vi "read_db_for_plot.vi"(6 "Small?":bool, 8 "error in (no error)":errorcluster, 9 "Limit no. of events":dbl=10000.0, 10 "Limited?":bool=TRUE, 11 "Constraints":T1 {"Estimate Quality" scale=0.0..5.0}) -> (0 "error out":errorcluster, 1 "Total Number of events":i64, 2 "Matching Events":i64, 3 "Dust Array":T2[](array[typedef]) {"File Location" items=["Unknown"=-5, "IDL Processing"=-4, "Writing from Queue"=-3, "Labview Files"=-2, "Retry Labview files"=-1, "Local Cache "=0, "Storage"=1]; "Estimate Source" items=["Any Source."=-2, "No Shot"=-1, "Basic Labview Estimate"=0, "IDL Estimate From Andrew"=1, "IDL Estimate From Tobin"=2, "Old Metadata"=3]}, 4 "Dust Info":cluster{"Density":dbl, "Name":string}[](array[cluster]))   [LabVIEW 2013]
uses:
  Public API/Query_Dust_Event.ctl
  Controls/Estimate_source.ctl
  Controls/File_location.ctl
  Controls/Constraints.ctl
  <vilib>/addons/database/Auxilliary.llb/DB Tools Cursor Type.ctl
  <userlib>/_OpenG.lib/array/array.llb/Remove Duplicates from 1D Array (String)__ogtk.vi
  <userlib>/_OpenG.lib/array/array.llb/Search 1D Array (String)__ogtk.vi
  <userlib>/_OpenG.lib/array/array.llb/Delete Elements from 1D Array (String)__ogtk.vi
  <vilib>/addons/database/Connection.llb/Conn Execute.vi
  <vilib>/addons/database/Recordset.llb/Rec Fetch Recordset Data (R).vi
  <vilib>/addons/database/Recordset.llb/Rec Destroy - Connection.vi
  <vilib>/addons/database/_DB Variant To Data/Database Variant To Data.xnode
  <vilib>/addons/database/NI_Database_API.lvlib
panel:
  out "Count Matching Events Syntax":string
  out "Count Events Syntax":string
  out "SQL Query Syntax":string
  # "Dust Event"
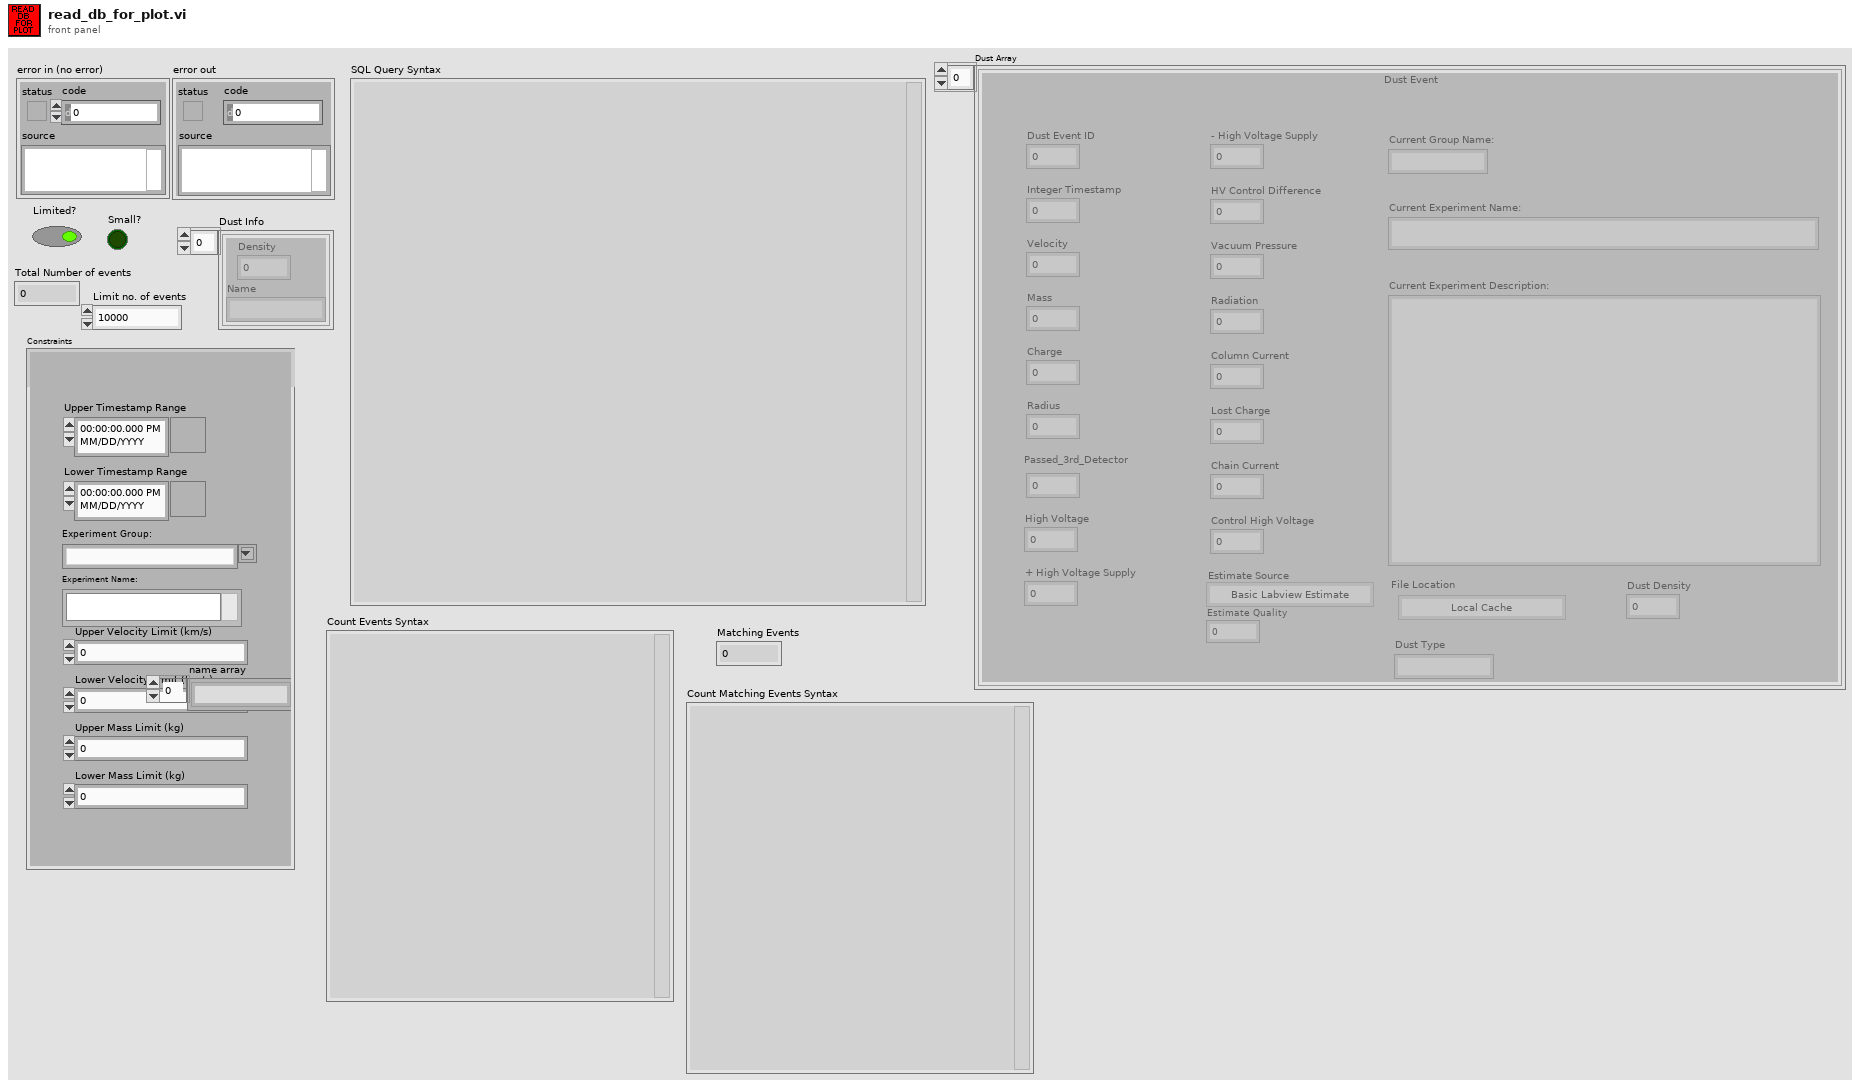
[diagram p1: front panel]
types:
  T1 = typedef "Constraints.ctl" = cluster{"Upper Timestamp Range":timestamp, "Lower Timestamp Range":timestamp, "Experiment Group:":string, "Experiment Name:":i32[], "Upper Velocity Limit (km/s)":dbl, "Lower Velocity Limit (km/s)":dbl, "Upper Mass Limit (kg)":dbl, "Lower Mass Limit (kg)":dbl, "name array":string[], "Estimate Quality":cluster{dbl, dbl}}
  T2 = typedef "Query_Dust_Event.ctl" = cluster{"Dust Event ID":i64, "Integer Timestamp":i64, "Velocity":sgl, "Mass":sgl, "Charge":sgl, "Radius":sgl, "Passed_3rd_Detector":i8, "High Voltage":sgl, "+ High Voltage Supply":sgl, "- High Voltage Supply":sgl, "HV Control Difference":sgl, "Vacuum Pressure":sgl, "Radiation":sgl, "Column Current":sgl, "Lost Charge":sgl, "Chain Current":sgl, "Control High Voltage":sgl, "Current Group Name:":string, "Current Experiment Name:":string, "Current Experiment Description:":string, "Estimate Source":T3, "Estimate Quality":sgl, "File Location":T4, "Dust Type":string, "Dust Density":sgl}
  T3 = typedef "Estimate_source.ctl" = i8
  T4 = typedef "File_location.ctl" = i8
  T5 = typedef "NI_Database_API.lvlib/DB Tools Cursor Type.ctl" = enum16{"forward-only", "keyset", "dynamic", "static"}
  T6 = typedef "NI_Database_API.lvlib/Conn ObjectReference.ctl" = refnum<k1>
  T7 = typedef "NI_Database_API.lvlib/Rec ObjectReference.ctl" = refnum<k1>
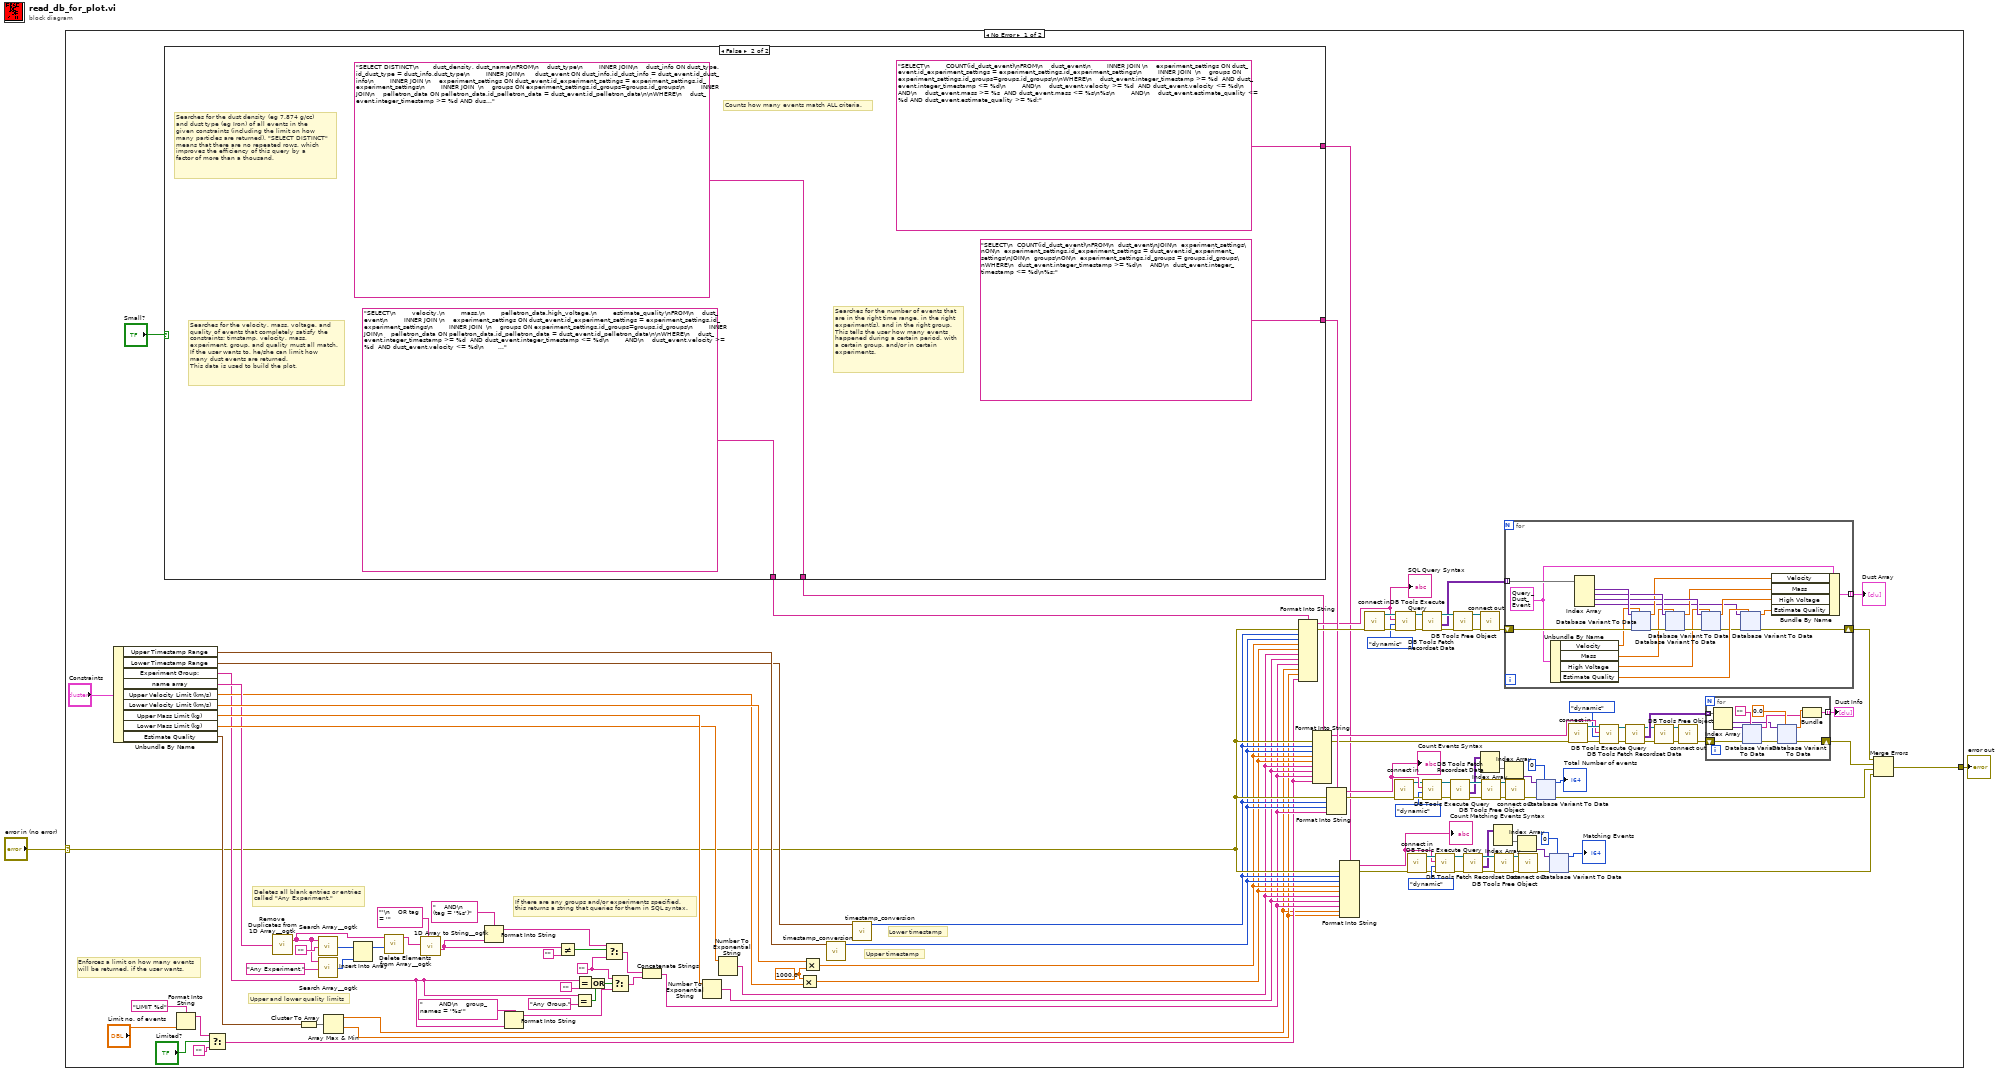
[diagram p0: block diagram]
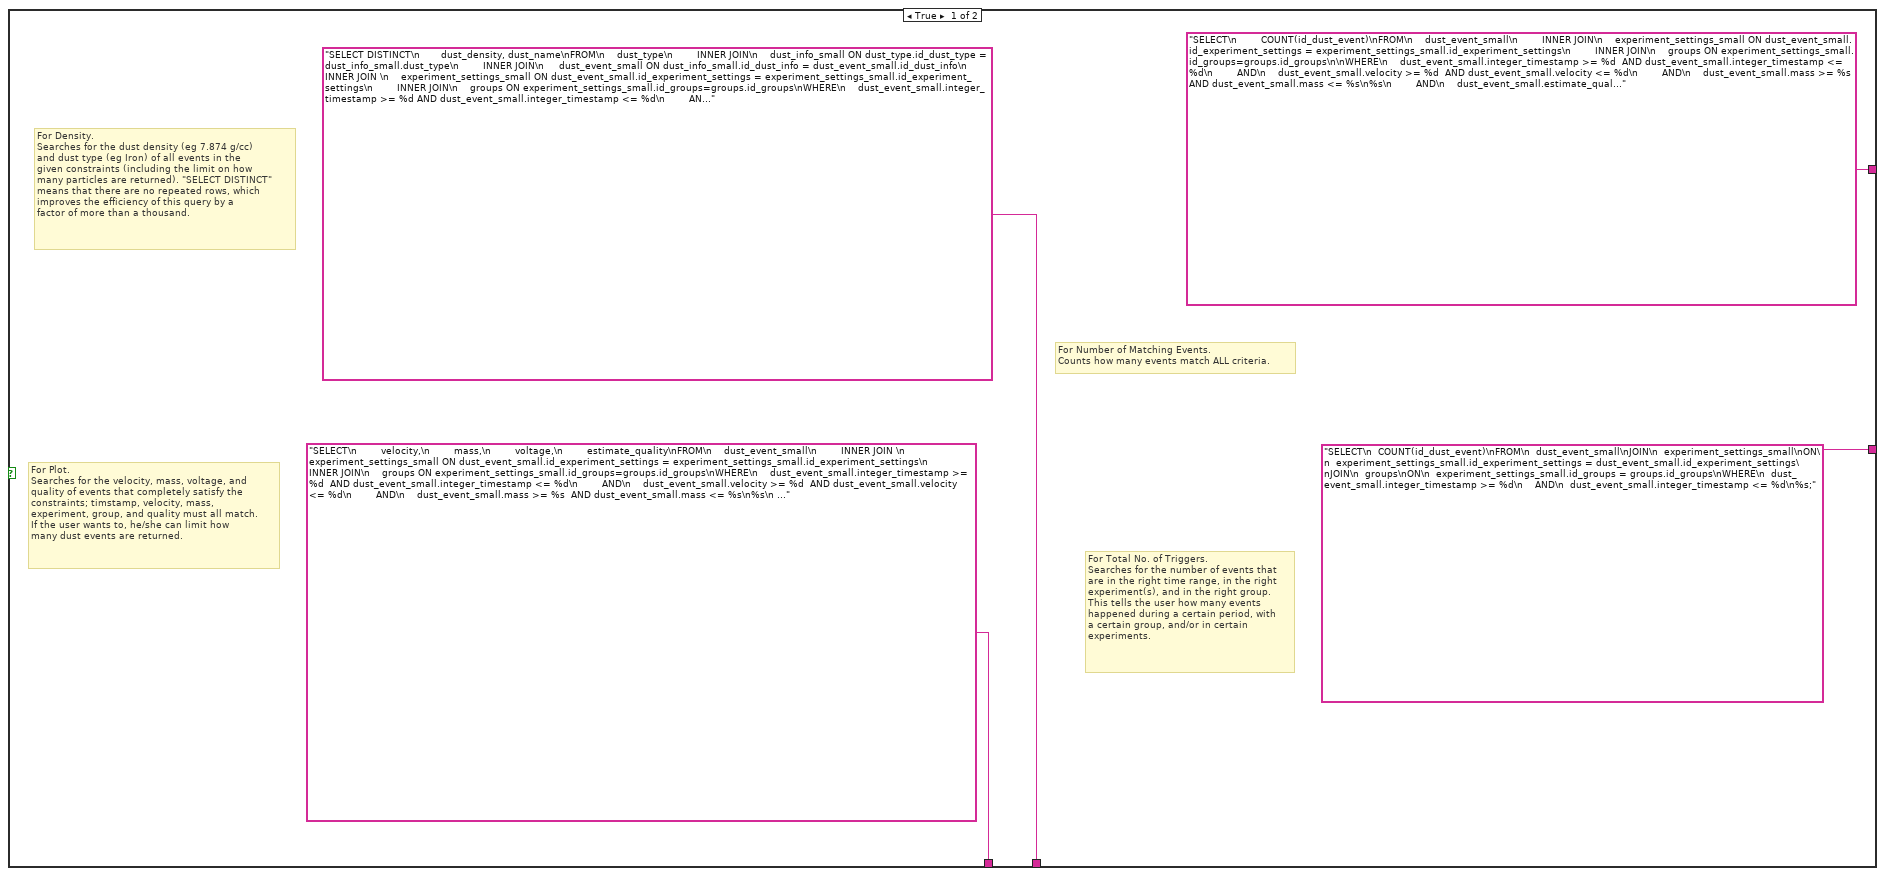
[diagram p2: hidden frame]
diagram:
  n1 = case shown="No Error" "error in (no error)" {
    selector: "error in (no error)" -> [w22 w421]
    tunnel: [w106 w421] -> w1
    frame No Error {
      w83 = 1000.0 ("y")
      w3 = ""
      # "Deletes all blank entries or entries\ncalled \"Any Experiment.\""
      # "Upper and lower quality limits"
      # "Upper timestamp"
      # "Lower timestamp"
      # "Enforces a limit on how many events\nwill be returned, if the user wants."
      # "If there are any groups and/or experiments specified,\nthis returns a string that queries for them in SQL syntax."
      n2 = Unbundle By Name("Constraints") -> ("Upper Timestamp Range"=w119:timestamp, "Lower Timestamp Range"=w55:timestamp, "Experiment Group:"=w47:string, "name array"=w57:string[], "Upper Velocity Limit (km/s)"=w54:dbl, "Lower Velocity Limit (km/s)"=w94:dbl, "Upper Mass Limit (kg)"=w114:dbl, "Lower Mass Limit (kg)"=w113:dbl, "Estimate Quality"=w82:cluster{dbl, dbl})
      n3 = case shown="False" "Small?" {
        tunnel: ["SELECT\n        velocity,\n        mass,\n        voltage,\n        estimate_quality\nFROM\n    dust_event_small\n        INNER JOIN \n    experiment_settings_small ON dust_event_small.id_experiment_settings = experiment_settings_small.id_experiment_settings\n        INNER JOIN\n    groups ON experiment_settings_small.id_groups=groups.id_groups\nWHERE\n    dust_event_small.integer_timestamp >= %d  AND dust_event_small.integer_timestamp <= %d\n        AND\n    dust_event_small.velocity >= %d  AND dust_event_small.velocity <= %d\n        AND\n    dust_event_small.mass >= %s  AND dust_event_small.mass <= %s\n%s\n        AND\n    dust_event_small.estimate_quality <= %d AND dust_event_small.estimate_quality >= %d\n        AND\n    dust_event_small.estimate_quality > 0\nORDER BY\n    id_dust_event DESC\n%s; " ("string") "SELECT\n        velocity,\n        mass,\n        pelletron_data.high_voltage,\n        estimate_quality\nFROM\n    dust_event\n        INNER JOIN \n    experiment_settings ON dust_event.id_experiment_settings = experiment_settings.id_experiment_settings\n        INNER JOIN  \n    groups ON experiment_settings.id_groups=groups.id_groups\n        INNER JOIN\n    pelletron_data ON pelletron_data.id_pelletron_data = dust_event.id_pelletron_data\n\nWHERE\n    dust_event.integer_timestamp >= %d  AND dust_event.integer_timestamp <= %d\n        AND\n    dust_event.velocity >= %d  AND dust_event.velocity <= %d\n        AND\n    dust_event.mass >= %s  AND dust_event.mass <= %s\n%s\n        AND\n    dust_event.estimate_quality <= %d AND dust_event.estimate_quality >= %d\n        AND\n    dust_event.estimate_quality > 0\nORDER BY\n    id_dust_event DESC\n%s; " ("string")] -> w110
        tunnel: ["SELECT\n  COUNT(id_dust_event)\nFROM\n  dust_event_small\nJOIN\n  experiment_settings_small\nON\n  experiment_settings_small.id_experiment_settings = dust_event_small.id_experiment_settings\nJOIN\n  groups\nON\n  experiment_settings_small.id_groups = groups.id_groups\nWHERE\n  dust_event_small.integer_timestamp >= %d\n    AND\n  dust_event_small.integer_timestamp <= %d\n%s;" ("SQL query") "SELECT\n  COUNT(id_dust_event)\nFROM\n  dust_event\nJOIN\n  experiment_settings\nON\n  experiment_settings.id_experiment_settings = dust_event.id_experiment_settings\nJOIN\n  groups\nON\n  experiment_settings.id_groups = groups.id_groups\nWHERE\n  dust_event.integer_timestamp >= %d\n    AND\n  dust_event.integer_timestamp <= %d\n%s;" ("SQL query")] -> w103
        tunnel: ["SELECT\n        COUNT(id_dust_event)\nFROM\n    dust_event_small\n        INNER JOIN\n    experiment_settings_small ON dust_event_small.id_experiment_settings = experiment_settings_small.id_experiment_settings\n        INNER JOIN\n    groups ON experiment_settings_small.id_groups=groups.id_groups\n\nWHERE\n    dust_event_small.integer_timestamp >= %d  AND dust_event_small.integer_timestamp <= %d\n        AND\n    dust_event_small.velocity >= %d  AND dust_event_small.velocity <= %d\n        AND\n    dust_event_small.mass >= %s  AND dust_event_small.mass <= %s\n%s\n        AND\n    dust_event_small.estimate_quality <= %d AND dust_event_small.estimate_quality >= %d;" ("string") "SELECT\n        COUNT(id_dust_event)\nFROM\n    dust_event\n        INNER JOIN \n    experiment_settings ON dust_event.id_experiment_settings = experiment_settings.id_experiment_settings\n        INNER JOIN  \n    groups ON experiment_settings.id_groups=groups.id_groups\n\nWHERE\n    dust_event.integer_timestamp >= %d  AND dust_event.integer_timestamp <= %d\n        AND\n    dust_event.velocity >= %d  AND dust_event.velocity <= %d\n        AND\n    dust_event.mass >= %s  AND dust_event.mass <= %s\n%s\n        AND\n    dust_event.estimate_quality <= %d AND dust_event.estimate_quality >= %d;" ("string")] -> w23
        tunnel: ["SELECT DISTINCT\n       dust_density, dust_name\nFROM\n    dust_type\n        INNER JOIN\n    dust_info_small ON dust_type.id_dust_type = dust_info_small.dust_type\n        INNER JOIN\n     dust_event_small ON dust_info_small.id_dust_info = dust_event_small.id_dust_info\n        INNER JOIN \n    experiment_settings_small ON dust_event_small.id_experiment_settings = experiment_settings_small.id_experiment_settings\n        INNER JOIN\n    groups ON experiment_settings_small.id_groups=groups.id_groups\nWHERE\n    dust_event_small.integer_timestamp >= %d AND dust_event_small.integer_timestamp <= %d\n        AND\n    dust_event_small.velocity >= %d AND dust_event_small.velocity <= %d\n        AND\n    dust_event_small.mass >= %s  AND dust_event_small.mass <= %s\n%s\nORDER BY\n    id_dust_event DESC\n%s; " ("string") "SELECT DISTINCT\n       dust_density, dust_name\nFROM\n    dust_type\n        INNER JOIN\n    dust_info ON dust_type.id_dust_type = dust_info.dust_type\n        INNER JOIN\n     dust_event ON dust_info.id_dust_info = dust_event.id_dust_info\n        INNER JOIN \n    experiment_settings ON dust_event.id_experiment_settings = experiment_settings.id_experiment_settings\n        INNER JOIN  \n    groups ON experiment_settings.id_groups=groups.id_groups\n        INNER JOIN\n    pelletron_data ON pelletron_data.id_pelletron_data = dust_event.id_pelletron_data\n\nWHERE\n    dust_event.integer_timestamp >= %d AND dust_event.integer_timestamp <= %d\n        AND\n    dust_event.velocity >= %d AND dust_event.velocity <= %d\n        AND\n    dust_event.mass >= %s  AND dust_event.mass <= %s\n%s\nORDER BY\n    id_dust_event DESC\n%s; " ("string")] -> w11
        frame True {
          # "For Number of Matching Events.\nCounts how many events match ALL criteria."
          # "For Density.\nSearches for the dust density (eg 7.874 g/cc)\nand dust type (eg Iron) of all events in the\ngiven constraints (including the limit on how\nmany particles are returned). \"SELECT DISTINCT\"\nmeans that there are no repeated rows, which\nimproves the efficiency of this query by a\nfactor of more than a thousand."
          # "For Plot.\nSearches for the velocity, mass, voltage, and\nquality of events that completely satisfy the\nconstraints; timstamp, velocity, mass,\nexperiment, group, and quality must all match.\nIf the user wants to, he/she can limit how\nmany dust events are returned."
          # "For Total No. of Triggers.\nSearches for the number of events that\nare in the right time range, in the right\nexperiment(s), and in the right group.\nThis tells the user how many events\nhappened during a certain period, with\na certain group, and/or in certain\nexperiments."
        }
        frame False {
          # "Counts how many events match ALL criteria."
          # "Searches for the dust density (eg 7.874 g/cc)\nand dust type (eg Iron) of all events in the\ngiven constraints (including the limit on how\nmany particles are returned). \"SELECT DISTINCT\"\nmeans that there are no repeated rows, which\nimproves the efficiency of this query by a\nfactor of more than a thousand."
          # "Searches for the velocity, mass, voltage, and\nquality of events that completely satisfy the\nconstraints; timstamp, velocity, mass,\nexperiment, group, and quality must all match.\nIf the user wants to, he/she can limit how\nmany dust events are returned. \nThis data is used to build the plot."
          # "Searches for the number of events that\nare in the right time range, in the right\nexperiment(s), and in the right group.\nThis tells the user how many events\nhappened during a certain period, with\na certain group, and/or in certain\nexperiments."
        }
      }
      n4 = Format Into String(format string="LIMIT %d", "Limit no. of events") -> (resulting string=w77:string)  [unwired: 2 in, 1 out]
      n5 = Select(t=w77, s="Limited?", f="") -> (s? t:f=w14:string)
      n6 = call-poly <userlib>:"Remove Duplicates from 1D Array__ogtk.vi"("Input Array"=w57) -> ("Output Array"=w8:string[])  [unwired: 1 out]
      n7 = Cluster To Array(cluster=w82) -> (array=w81:dbl[])
      n8 = call-poly <userlib>:"Search Array__ogtk.vi"("Array"=w8, "Element Data"="") -> ("Indices of Elements"=w50:i32[])  [unwired: 7 in]
      n9 = call-poly <userlib>:"Search Array__ogtk.vi"("Array"=w8, "Element Data"="Any Experiment.") -> ("Indices of Elements"=w6:i32[])  [unwired: 7 in]
      n10 = Array Max & Min(array=w81) -> (max value=w12:dbl, min value=w13:dbl)  [unwired: 2 out]
      n11 = Insert Into Array(array=w50, new element=w6) -> (w7:i32[])  [unwired: 1 in]
      n12 = call-poly <userlib>:"Delete Elements from Array__ogtk.vi"("indices"=w7, "array"=w8) -> ("array w/ subset deleted"=w49:string[])  [unwired: 8 in, 1 out]
      n13 = call <userlib>:"1D Array to String__ogtk.vi"("delimiter (Tab)"="'\n    OR tag = '", "Array of Strings"=w49) -> ("delimited string"=w42:string)  [unwired: 9 in]
      n14 = Format Into String(format string="    AND\n  (tag = '%s')" ("string"), w42) -> (resulting string=w4:string)  [unwired: 2 in, 1 out]
      n15 = Format Into String(format string="        AND\n    group_names = '%s'" ("string"), w47) -> (resulting string=w116:string)  [unwired: 2 in, 1 out]
      n16 = Not Equal?(x=w42, y="") -> (x != y?=w5:bool)
      n17 = Equal?(x=w47, y="Any Group.") -> (x = y?=w48:bool)
      n18 = Equal?(x=w47, y="") -> (x = y?=w44:bool)
      n19 = Or(x=w44, y=w48) -> (x .or. y?=w45:bool)
      n20 = Select(t=w4, s=w5, f=w3) -> (s? t:f=w121:string)
      n21 = Select(t=w3, s=w45, f=w116) -> (s? t:f=w120:string)
      n22 = Concatenate Strings(w121, w120) -> (w15:string)
      n23 = Number To Exponential String(number=w114) -> (E-format string=w16:string)  [unwired: 3 in]
      n24 = Number To Exponential String(number=w113) -> (E-format string=w17:string)  [unwired: 3 in]
      n25 = Multiply(x=w83, y=w54) -> (x*y=w18:dbl)
      n26 = Multiply(x=w94, y=w83) -> (x*y=w19:dbl)
      n27 = call "timestamp_conversion.vi"("Time Stamp"=w119) -> ("Integer Time"=w20:i64)  [unwired: 8 in, 1 out]
      n28 = call "timestamp_conversion.vi"("Time Stamp"=w55) -> ("Integer Time"=w21:i64)  [unwired: 8 in, 1 out]
      n29 = Format Into String(format string=w110, error in=w22, w21, w20, w19, w18, w17, w16, w15, w12, w13, w14) -> (resulting string=w53:string, error out=w109:errorcluster)  [unwired: 1 in]
      "SQL Query Syntax" <- w53
      n30 = Format Into String(format string=w11, error in=w22, w21, w20, w19, w18, w17, w16, w15, w14) -> (resulting string=w91:string, error out=w93:errorcluster)  [unwired: 1 in]
      n31 = Format Into String(format string=w103, error in=w22, w21, w20, w15) -> (resulting string=w102:string, error out=w69:errorcluster)  [unwired: 1 in]
      "Count Events Syntax" <- w102
      n32 = Format Into String(format string=w23, error in=w22, w21, w20, w19, w18, w17, w16, w15, w12, w13) -> (resulting string=w27:string, error out=w35:errorcluster)  [unwired: 1 in]
      "Count Matching Events Syntax" <- w27
      n33 = call "connect in.vi"("error in (no error)"=w109) -> ("error out"=w97:errorcluster, "Database Connection"=w107:T6)  [unwired: 6 in, 1 out]
      n34 = call "connect in.vi"("error in (no error)"=w69) -> ("error out"=w68:errorcluster, "Database Connection"=w96:T6)  [unwired: 6 in, 1 out]
      n35 = call-poly <vilib>:"DB Tools Execute Query.vi"("error in (no error)"=w97, "cursor type"=DB_Tools_Cursor_Type."dynamic", "SQL query"=w53, "connection reference"=w107) -> ("error out"=w112:errorcluster, "recordset reference"=w111:T7)  [unwired: 4 in]
      n36 = call "connect in.vi"("error in (no error)"=w35) -> ("error out"=w36:errorcluster, "Database Connection"=w33:T6)  [unwired: 6 in, 1 out]
      n37 = call-poly <vilib>:"DB Tools Fetch Recordset Data.vi"("error in (no error)"=w112, "recordset reference"=w111) -> ("error out"=w73:errorcluster, "recordset data"=w123:variant[][], "recordset reference out"=w125:T7)  [unwired: 3 in]
      n38 = call-poly <vilib>:"DB Tools Execute Query.vi"("error in (no error)"=w68, "cursor type"=DB_Tools_Cursor_Type."dynamic", "SQL query"=w102, "connection reference"=w96) -> ("error out"=w108:errorcluster, "recordset reference"=w105:T7)  [unwired: 4 in]
      n39 = call-poly <vilib>:"DB Tools Execute Query.vi"("error in (no error)"=w36, "cursor type"=DB_Tools_Cursor_Type."dynamic", "SQL query"=w27, "connection reference"=w33) -> ("error out"=w28:errorcluster, "recordset reference"=w29:T7)  [unwired: 4 in]
      n40 = call-poly <vilib>:"DB Tools Fetch Recordset Data.vi"("error in (no error)"=w108, "recordset reference"=w105) -> ("error out"=w66:errorcluster, "recordset data"=w101:variant[][], "recordset reference out"=w104:T7)  [unwired: 3 in]
      n41 = call-poly <vilib>:"DB Tools Free Object.vi"("error in (no error)"=w73, "recordset reference"=w125) -> ("error out"=w74:errorcluster, "connection reference"=w124:T6)  [unwired: 8 in]
      n42 = call-poly <vilib>:"DB Tools Fetch Recordset Data.vi"("error in (no error)"=w28, "recordset reference"=w29) -> ("error out"=w38:errorcluster, "recordset data"=w26:variant[][], "recordset reference out"=w30:T7)  [unwired: 3 in]
      n43 = call "connect out.vi"("error in (no error)"=w74, "connection reference"=w124) -> ("error out"=w72:errorcluster)  [unwired: 9 in]
      n44 = Index Array(array=w101) -> (element=w100:variant[])  [unwired: 2 in]
      n45 = call-poly <vilib>:"DB Tools Free Object.vi"("error in (no error)"=w66, "recordset reference"=w104) -> ("error out"=w67:errorcluster, "connection reference"=w95:T6)  [unwired: 8 in]
      n46 = Index Array(array=w26) -> (element=w31:variant[])  [unwired: 2 in]
      n47 = call-poly <vilib>:"DB Tools Free Object.vi"("error in (no error)"=w38, "recordset reference"=w30) -> ("error out"=w37:errorcluster, "connection reference"=w34:T6)  [unwired: 8 in]
      n48 = for {
        tunnel: w123 -> [w292] mode=indexing
        shift-right: [w284] -> w71
        shift-left: w72 -> [w291]
        tunnel: [w283] -> w122 mode=indexing
        w289 = T2 {"Dust Event ID"=0, "Integer Timestamp"=0, "Velocity"=0.0, "Mass"=0.0, "Charge"=0.0, "Radius"=0.0, "Passed_3rd_Detector"=0, "High Voltage"=0.0, "+ High Voltage Supply"=0.0, "- High Voltage Supply"=0.0, "HV Control Difference"=0.0, "Vacuum Pressure"=0.0, "Radiation"=0.0, "Column Current"=0.0, "Lost Charge"=0.0, "Chain Current"=0.0, "Control High Voltage"=0.0, "Current Group Name:"="", "Current Experiment Name:"="", "Current Experiment Description:"="", "Estimate Source"=0, "Estimate Quality"=0.0, "File Location"=0, "Dust Type"="", "Dust Density"=0.0} ("Cluster")
        n49 = Unbundle By Name(w289) -> ("Velocity"=w282:sgl, "Mass"=w280:sgl, "High Voltage"=w278:sgl, "Estimate Quality"=w276:sgl)
        n50 = Index Array(array=w292) -> (element #1=w290:variant, element #2=w288:variant, element #3=w286:variant, element #4=w273:variant)  [unwired: 4 in]
        n51 = xnode "Database Variant To Data"("database variant"=w290, "error in"=w291, "type"=w282) -> ("data"=w281:sgl, "error out"=w287:errorcluster)
        n52 = xnode "Database Variant To Data"("database variant"=w288, "error in"=w287, "type"=w280) -> ("data"=w279:sgl, "error out"=w285:errorcluster)
        n53 = xnode "Database Variant To Data"("database variant"=w286, "error in"=w285, "type"=w278) -> ("data"=w277:sgl, "error out"=w274:errorcluster)
        n54 = xnode "Database Variant To Data"("database variant"=w273, "error in"=w274, "type"=w276) -> ("data"=w275:sgl, "error out"=w284:errorcluster)
        n55 = Bundle By Name(cluster=w289, "Velocity"=w281, "Mass"=w279, "High Voltage"=w277, "Estimate Quality"=w275) -> (w283:T2)
      }
      "Dust Array" <- w122
      n56 = Index Array(array=w100) -> (element=w99:variant)  [unwired: 1 in]
      n57 = call "connect out.vi"("error in (no error)"=w67, "connection reference"=w95) -> ("error out"=w65:errorcluster)  [unwired: 9 in]
      n58 = Index Array(array=w31) -> (element=w32:variant)  [unwired: 1 in]
      n59 = call "connect out.vi"("error in (no error)"=w37, "connection reference"=w34) -> ("error out"=w39:errorcluster)  [unwired: 9 in]
      n60 = xnode "Database Variant To Data"("database variant"=w99, "error in (no error)"=w65, "type"=0) -> ("data"=→"Total Number of events":i32, "error out"=w64:errorcluster)
      n61 = xnode "Database Variant To Data"("database variant"=w32, "error in (no error)"=w39, "type"=0) -> ("data"=→"Matching Events":i32, "error out"=w25:errorcluster)
      n62 = call "connect in.vi"("error in (no error)"=w93) -> ("error out"=w84:errorcluster, "Database Connection"=w92:T6)  [unwired: 6 in, 1 out]
      n63 = call-poly <vilib>:"DB Tools Execute Query.vi"("error in (no error)"=w84, "cursor type"=DB_Tools_Cursor_Type."dynamic", "SQL query"=w91, "connection reference"=w92) -> ("error out"=w89:errorcluster, "recordset reference"=w90:T7)  [unwired: 4 in]
      n64 = call-poly <vilib>:"DB Tools Fetch Recordset Data.vi"("error in (no error)"=w89, "recordset reference"=w90) -> ("error out"=w63:errorcluster, "recordset data"=w88:variant[][], "recordset reference out"=w86:T7)  [unwired: 3 in]
      n65 = call-poly <vilib>:"DB Tools Free Object.vi"("error in (no error)"=w63, "recordset reference"=w86) -> ("error out"=w70:errorcluster, "connection reference"=w85:T6)  [unwired: 8 in]
      n66 = call "connect out.vi"("error in (no error)"=w70, "connection reference"=w85) -> ("error out"=w62:errorcluster)  [unwired: 9 in]
      n67 = for {
        tunnel: w88 -> [w176] mode=indexing
        shift-right: [w166] -> w61
        shift-left: w62 -> [w168]
        tunnel: [w170] -> w87 mode=indexing
        n68 = Index Array(array=w176) -> (element #1=w169:variant, element #2=w175:variant)  [unwired: 2 in]
        n69 = xnode "Database Variant To Data"("database variant"=w175, "error in (no error)"=w168, "type"="") -> ("data"=w171:string, "error out"=w167:errorcluster)
        n70 = xnode "Database Variant To Data"("database variant"=w169, "error in (no error)"=w167, "type"=0.0) -> ("data"=w172:dbl, "error out"=w166:errorcluster)
        n71 = Bundle("data"=w172, "data"=w171) -> (w170:cluster{"data":dbl, "data":string})  [unwired: 1 in]
      }
      "Dust Info" <- w87
      n72 = Merge Errors(w71, w61, w64, w25) -> (w106:errorcluster)
    }
    frame Error {
    }
  }
  "error out" <- w1
